vi "Plot grid style TO.vi"(10 "Grid Colors:Minor Color":u32(colorbox) caption="Minor grid", 11 "Grid Colors:Major Color":u32(colorbox) caption="Major grid") -> (3 "Grid Style":T1)   [LabVIEW 2021, in "RocketPlot.lvlib"]
uses:
  RocketPlot.lvlib
  horiz grid/plot horizontal grid pic ring.ctl
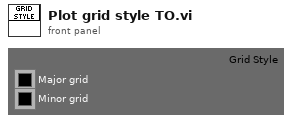
[diagram p1: front panel]
types:
  T1 = typedef "RocketPlot.lvlib/plot horizontal grid pic ring.ctl" = u16
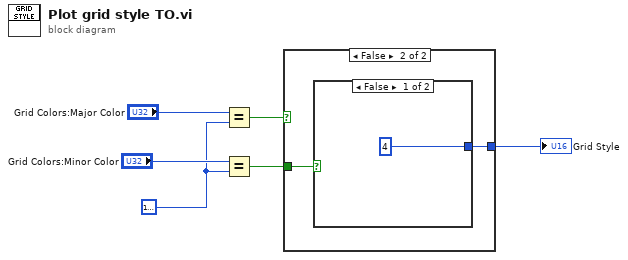
[diagram p0: block diagram]
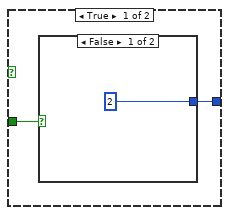
[diagram p2: hidden frame]
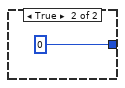
[diagram p3: hidden frame]
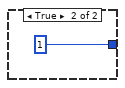
[diagram p4: hidden frame]
diagram:
  w4 = u32 16777216
  n1 = Equal?(x="Grid Colors:Major Color", y=w4) -> (x = y?=w3:bool)
  n2 = Equal?(x="Grid Colors:Minor Color", y=w4) -> (x = y?=w2:bool)
  n3 = case shown="False" w3 {
    tunnel: w2 -> [w8 w12]
    tunnel: [w7 w11] -> w1
    frame True {
      n4 = case shown="False" w8 {
        tunnel: [2 0] -> w7
        frame False {
        }
        frame True {
        }
      }
    }
    frame False {
      n5 = case shown="False" w12 {
        tunnel: [4 1] -> w11
        frame False {
        }
        frame True {
        }
      }
    }
  }
  "Grid Style" <- w1
